vi "Get Tx UDP Section and Channels.vi"(8 "error in":errorcluster, 10 "option":u16(ring) items=["Find VLs", "Find Parameters"], 11 "custom device ref in":T1 format="%.0x") -> (0 "error out":errorcluster, 1 "Tx UDP channel refs out":T1[](array[typedef]) format="%.0x", 2 "Tx UDP section ref out":T1 format="%.0x", 3 "custom device ref out":T1 format="%.0x", 4 "channels found?":bool, 6 "session found?":bool)   [LabVIEW 2020, in "AIM ARINC 664 Scripting.lvlib"]
uses:
  AIM ARINC 664 Scripting.lvlib
  <vilib>/NI VeriStand/Custom Device API/Custom Device Item Ref.ctl
  Constants.vi
  <vilib>/NI VeriStand/Custom Device API/Custom Device API.lvlib
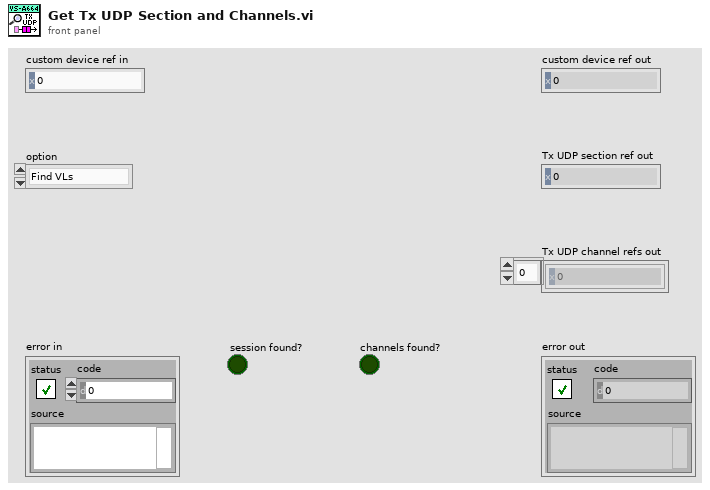
[diagram p1: front panel]
types:
  T1 = typedef "Custom Device API.lvlib/Custom Device Item Ref.ctl" = u64
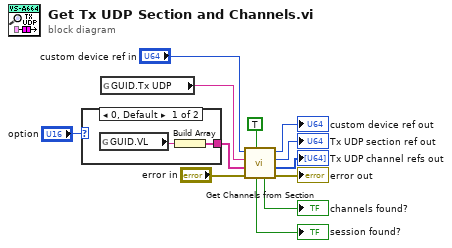
[diagram p0: block diagram]
diagram:
  n1 = case shown="0, Default" "option" {
    tunnel: [w13 _] -> w5
    frame 0, Default {
      n2 = global read "Constants.vi" "GUID.VL"() -> (w14:string)
      n3 = Build Array(w14) -> (w13:string[])
    }
    frame 1 {
    }
  }
  n4 = global read "Constants.vi" "GUID.Tx UDP"() -> (w3:string)
  n5 = call "Get Channels from Section.vi"("channel by GUID"=TRUE ("Channels by GUID"), "error in"="error in", "channel array names"=w5, "GUID section"=w3, "custom device ref in"="custom device ref in") -> ("error out"=→"error out":errorcluster, "channel array refs out"=→"Tx UDP channel refs out":T1[], "section ref out"=→"Tx UDP section ref out":T1, "custom device ref out"=→"custom device ref out":T1, "all channels found?"=→"channels found?":bool, "session found?"=→"session found?":bool)  [unwired: 1 in]
